vi "r-songstructure.vi"(11 "Song structure":T1 {"Outro %" format="%#_13g"; "Solo %" format="%#_13g"; "Bridge %" format="%#_13g"; "Intro %" format="%#_13g"}) -> (3 "shuffled array":string[](array[string]))   [LabVIEW 2019]
uses:
  song-structure.ctl
  <vilib>/numeric/Random Number (Range) I64.vi
  7d7bcb52-9932-4f12-92ae-012c9415b29b.vi
  <vilib>/numeric/sub_Random U32.vi
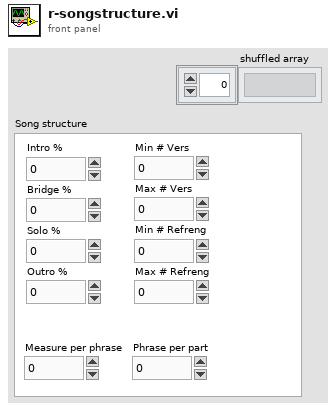
[diagram p1: front panel]
types:
  T1 = typedef "song-structure.ctl" = cluster{"Intro %":dbl, "Bridge %":dbl, "Solo %":dbl, "Outro %":dbl, "Min # Vers":i32, "Max # Vers":i32, "Min # Refreng":i32, "Max # Refreng":i32, "Measure per phrase":i32, "Phrase per part":i32}
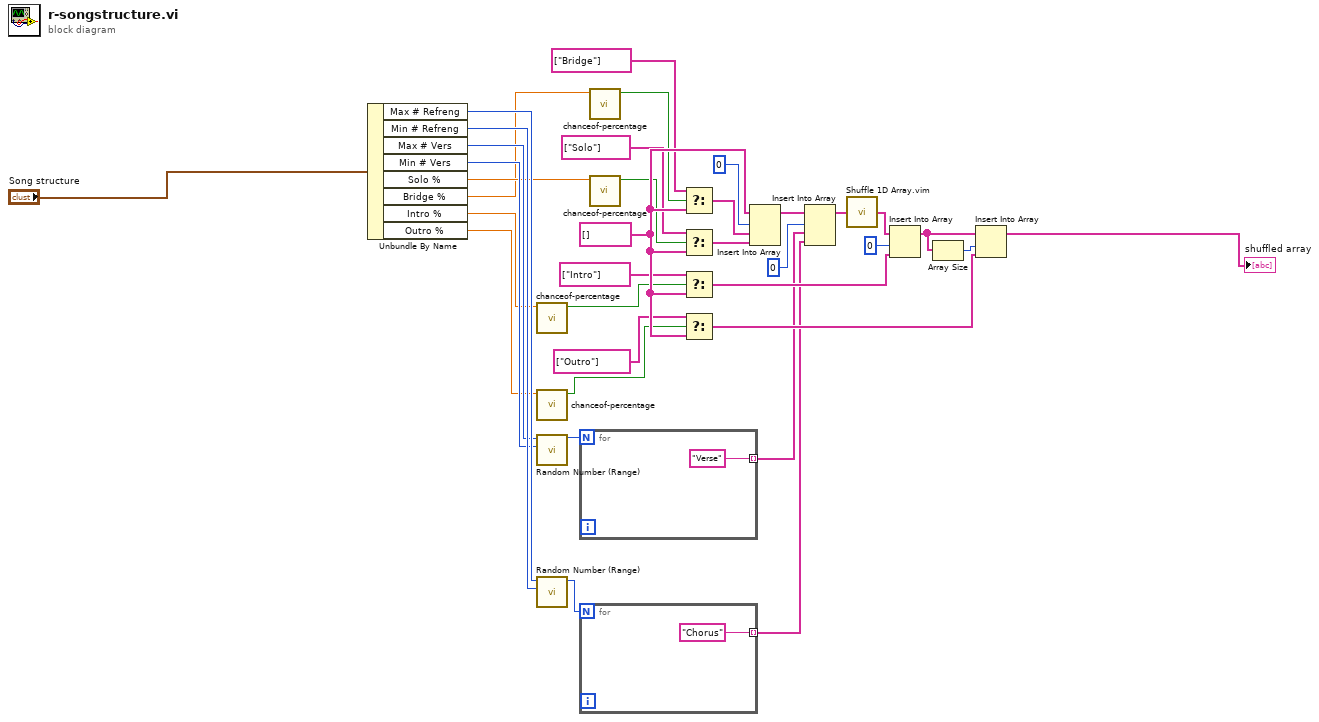
[diagram p0: block diagram]
diagram:
  w25 = string[] []
  n1 = Unbundle By Name("Song structure") -> ("Max # Refreng"=w35:i32, "Min # Refreng"=w34:i32, "Max # Vers"=w33:i32, "Min # Vers"=w32:i32, "Solo %"=w30:dbl, "Bridge %"=w29:dbl, "Intro %"=w28:dbl, "Outro %"=w31:dbl)
  n2 = call "chanceof-percentage.vi"("Chance of Intro"=w28) -> ("Present"=w3:bool)  [unwired: 10 in]
  n3 = call "chanceof-percentage.vi"("Chance of Intro"=w31) -> ("Present"=w23:bool)  [unwired: 10 in]
  n4 = call-poly <vilib>:"Random Number (Range).vi"("lower bound (-100)"=w32, "upper bound (100)"=w33) -> ("number"=w5:i64)  [unwired: 9 in]
  n5 = call-poly <vilib>:"Random Number (Range).vi"("lower bound (-100)"=w34, "upper bound (100)"=w35) -> ("number"=w4:i64)  [unwired: 9 in]
  n6 = for {
    N: w5 -> [_]
    tunnel: ["Verse"] -> w15 mode=indexing
  }
  n7 = for {
    N: w4 -> [_]
    tunnel: ["Chorus"] -> w16 mode=indexing
  }
  n8 = call "chanceof-percentage.vi"("Chance of Intro"=w29) -> ("Present"=w6:bool)  [unwired: 10 in]
  n9 = call "chanceof-percentage.vi"("Chance of Intro"=w30) -> ("Present"=w8:bool)  [unwired: 10 in]
  n10 = Select(t=string[] ["Bridge"], s=w6, f=w25) -> (s? t:f=w10:string[])
  n11 = Select(t=string[] ["Solo"], s=w8, f=w25) -> (s? t:f=w11:string[])
  n12 = Select(t=string[] ["Intro"], s=w3, f=w25) -> (s? t:f=w20:string[])
  n13 = Select(t=string[] ["Outro"], s=w23, f=w25) -> (s? t:f=w26:string[])
  n14 = Insert Into Array(array=w25, index=0, new element #1=w10, new element #2=w11) -> (w13:string[])
  n15 = Insert Into Array(array=w13, index=0, new element #1=w15, new element #2=w16) -> (w17:string[])
  n16 = call "Shuffle 1D Array.vim"("array"=w17) -> ("shuffled array"=w18:string[])  [unwired: 4 in]
  n17 = Insert Into Array(array=w18, index=0, new element=w20) -> (w22:string[])
  n18 = Array Size(array=w22) -> (size(s)=w21:i32)
  n19 = Insert Into Array(array=w22, index=w21, new element=w26) -> (→"shuffled array":string[])
